vi "Team Selection.vi"() -> ()   [LabVIEW 2020]
panel:
  out "4":string[](array[string])=["Captain 4"]
  out "3":string[](array[string])=["Captain 3"]
  out "2":string[](array[string])=["Captain 2"]
  out "1":string[](array[string])=["Captain 1"]
  in  "Names":string[](array[string])
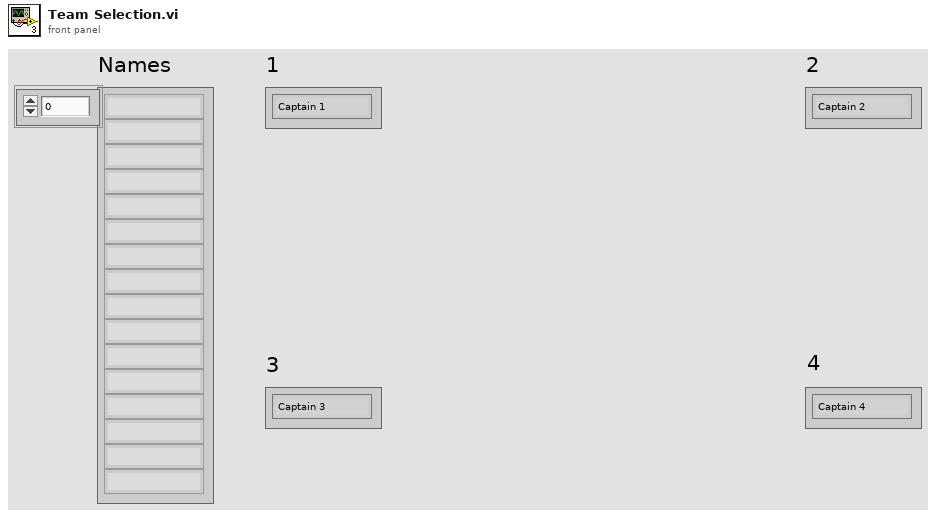
[diagram p1: front panel]
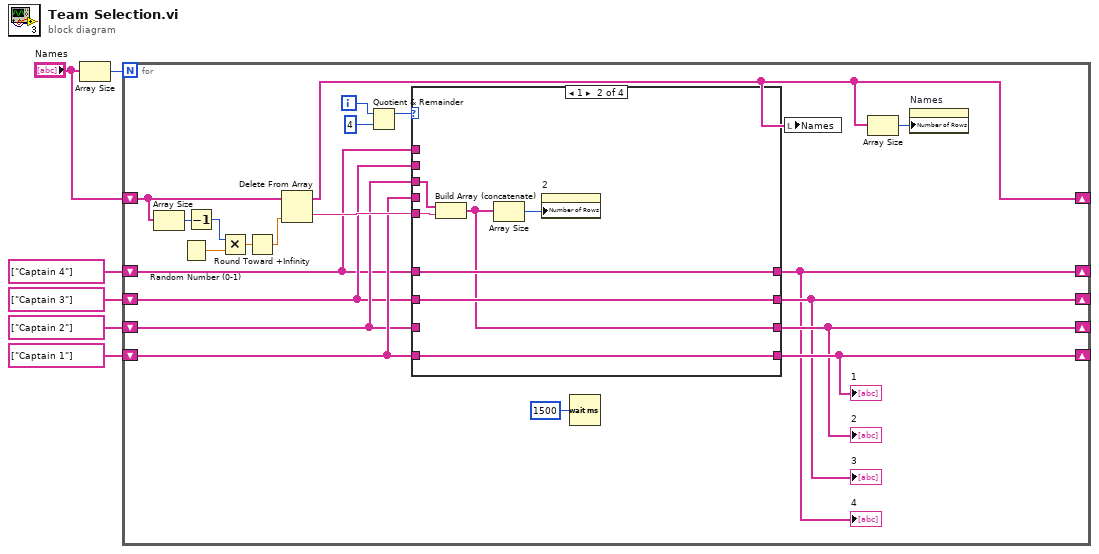
[diagram p0: block diagram]
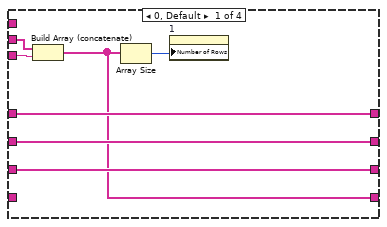
[diagram p2: hidden frame]
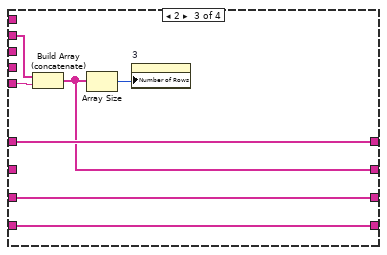
[diagram p3: hidden frame]
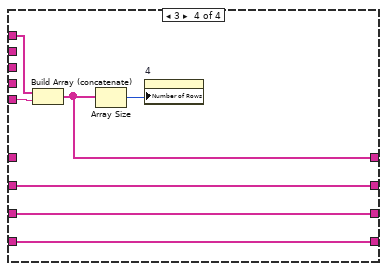
[diagram p4: hidden frame]
diagram:
  n1 = Array Size(array="Names") -> (size(s)=w6:i32)
  n2 = for {
    N: w6 -> [_]
    shift-right: [w15] -> _
    shift-left: string[] ["Captain 4"] -> [w19]
    shift-right: [w16] -> _
    shift-left: string[] ["Captain 3"] -> [w20]
    shift-right: [w17] -> _
    shift-left: string[] ["Captain 2"] -> [w21]
    shift-right: [w18] -> _
    shift-left: string[] ["Captain 1"] -> [w22]
    shift-right: [w8] -> _
    shift-left: "Names" -> [w13]
    i -> [w27]
    n3 = Array Size(array=w13) -> (size(s)=w12:i32)
    n4 = Random Number (0-1)() -> (number: 0 to 1=w14:dbl)
    n5 = Decrement(x=w12) -> (x-1=w10:i32)
    n6 = Multiply(x=w10, y=w14) -> (x*y=w11:dbl)
    n7 = Round Toward +Infinity(x=w11) -> (ceil(x): smallest int >= x=w9:dbl)
    n8 = Delete From Array(array=w13, index=w9) -> (deleted portion=w24:string, array with subset deleted=w8:string[])  [unwired: 1 in]
    n9 = Quotient & Remainder(x=w27, y=4) -> (x-y*floor(x/y)=w25:i32)  [unwired: 1 out]
    n10 = case shown="1" w25 {
      tunnel: w24 -> [w30 w37 w44 w51]
      tunnel: [w34 w41 w48 w50] -> w15
      tunnel: w19 -> [_ _ _ w55]
      tunnel: [w33 w40 w43 w54] -> w16
      tunnel: w19 -> [w34 w41 w48 _]
      tunnel: [w32 w36 w47 w53] -> w17
      tunnel: w20 -> [w33 w40 _ w54]
      tunnel: [w29 w39 w46 w52] -> w18
      tunnel: w21 -> [w32 _ w47 w53]
      tunnel: w22 -> [_ w39 w46 w52]
      tunnel: w20 -> [_ _ w45 _]
      tunnel: w21 -> [_ w38 _ _]
      tunnel: w22 -> [w31 _ _ _]
      frame 0, Default {
        n11 = Build Array (concatenate)(w31, w30) -> (w29:string[])
        n12 = Array Size(array=w29) -> (size(s)=w28:i32)
        n13 = property on="1" class="Arr (strict)"("Number of Rows"=w28) -> ()  [unwired: 2 in, 2 out]
      }
      frame 1 {
        n14 = Build Array (concatenate)(w38, w37) -> (w36:string[])
        n15 = Array Size(array=w36) -> (size(s)=w35:i32)
        n16 = property on="2" class="Arr (strict)"("Number of Rows"=w35) -> ()  [unwired: 2 in, 2 out]
      }
      frame 2 {
        n17 = Build Array (concatenate)(w45, w44) -> (w43:string[])
        n18 = Array Size(array=w43) -> (size(s)=w42:i32)
        n19 = property on="3" class="Arr (strict)"("Number of Rows"=w42) -> ()  [unwired: 2 in, 2 out]
      }
      frame 3 {
        n20 = Build Array (concatenate)(w55, w51) -> (w50:string[])
        n21 = Array Size(array=w50) -> (size(s)=w49:i32)
        n22 = property on="4" class="Arr (strict)"("Number of Rows"=w49) -> ()  [unwired: 2 in, 2 out]
      }
    }
    "1" <- w18
    "2" <- w17
    "3" <- w16
    "4" <- w15
    n23 = Wait (ms)(milliseconds to wait=u32 1500) -> ()  [unwired: 1 out]
    n24 = local write "Names"(w8) -> ()
    n25 = Array Size(array=w8) -> (size(s)=w7:i32)
    n26 = property on="Names" class="Arr (strict)"("Number of Rows"=w7) -> ()  [unwired: 2 in, 2 out]
  }
